vi "Update Configuration.vi"(8 "error in (no error)":errorcluster, 10 "ConfigDTO":refnum<class "ConfigDTO.lvclass">, 11 "MainActor in":refnum<class "MainActor.lvclass">) -> (0 "error out":errorcluster, 3 "MainActor out":refnum<class "MainActor.lvclass">)   [LabVIEW 2025, in "MainActor.lvlib" / "MainActor.lvclass"]
uses:
  MainActor.lvclass
  DataTransisionObjects/ConfigDTO/ConfigDTO.lvclass
  MainActor.lvclass/MainActor.ctl
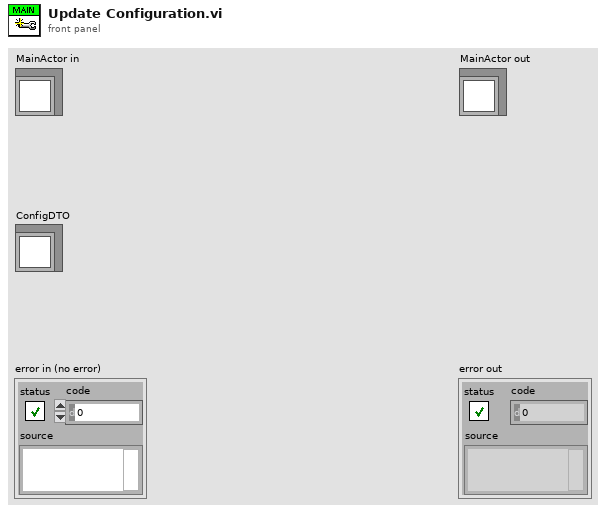
[diagram p1: front panel]
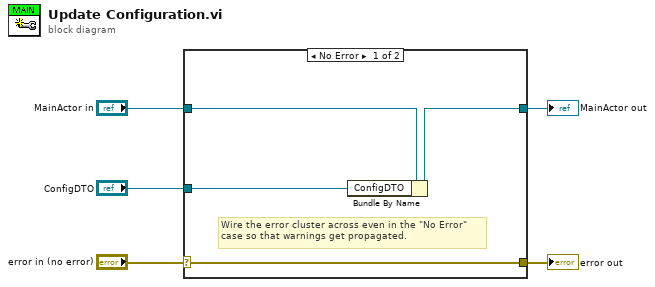
[diagram p0: block diagram]
diagram:
  n1 = case shown="No Error" "error in (no error)" {
    selector: "error in (no error)" -> [w8 w11]
    tunnel: [w8 w11] -> w4
    tunnel: [w7 w10] -> w2
    tunnel: "MainActor in" -> [w9 w10]
    tunnel: "ConfigDTO" -> [w6 _]
    frame No Error {
      # "Wire the error cluster across even in the \"No Error\"\ncase so that warnings get propagated."
      n2 = Bundle By Name(cluster=w9, "ConfigDTO"=w6) -> (w7:refnum<class "MainActor.lvclass">)
    }
    frame Error {
    }
  }
  "error out" <- w4
  "MainActor out" <- w2
